vi "Create UI_Generator_config.vi"(8 "error in (no error)":errorcluster, 10 "system":refnum<class "multichannel-lockin.lvclass">, 11 "UI_Generator_Config":refnum<class "UI_Generator_Config.lvclass">) -> (0 "error out":errorcluster, 3 "UI_Generator_Config":refnum<class "UI_Generator_Config.lvclass">)   [LabVIEW 2019, in "UI_Generator_Config.lvclass"]
uses:
  UI_Generator_Config.lvclass
  C:/Program Files (x86)/National Instruments/LabVIEW 2019/vi.lib/JKI/JKI SMO/SMO/SMO.lvclass
  lockin/multichannel-lockin.lvclass
  UI_Generator_Config.lvclass/UI_Generator_Config.ctl
  <vilib>/JKI/JKI SMO/SMO/SMO.lvclass
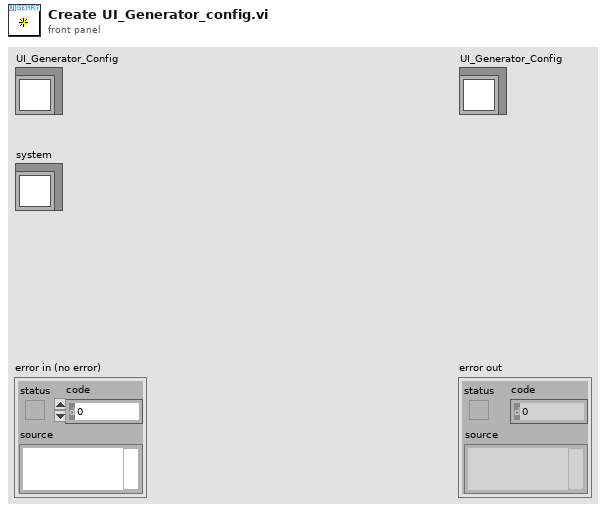
[diagram p1: front panel]
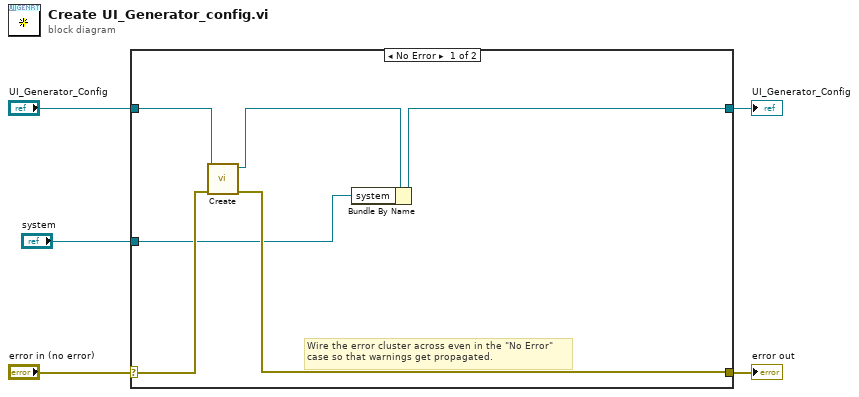
[diagram p0: block diagram]
diagram:
  n1 = case shown="No Error" "error in (no error)" {
    selector: "error in (no error)" -> [w11 w13]
    tunnel: [w10 w13] -> w4
    tunnel: "UI_Generator_Config" -> [w9 w12]
    tunnel: [w7 w12] -> w2
    tunnel: "system" -> [w6 _]
    frame No Error {
      # "Wire the error cluster across even in the \"No Error\"\ncase so that warnings get propagated."
      n2 = call <vilib>:"Create.vi"("error in (no error)"=w11, "SMO"=w9) -> ("error out"=w10:errorcluster, "SMO out"=w8:refnum<class "UI_Generator_Config.lvclass">)  [unwired: 7 in, 1 out]
      n3 = Bundle By Name(cluster=w8, "system"=w6) -> (w7:refnum<class "UI_Generator_Config.lvclass">)
    }
    frame Error {
    }
  }
  "error out" <- w4
  "UI_Generator_Config" <- w2
